vi "get_pixel_number.vi"(11 "Device details":T1={"Device label"="", "Experiment Variable"="", "Variable Value"="", "Pixel"=enum."1"}) -> (2 "Pixel string":string, 3 "Pixel":i32)   [LabVIEW 2018]
uses:
  typedefs/device_details.ctl
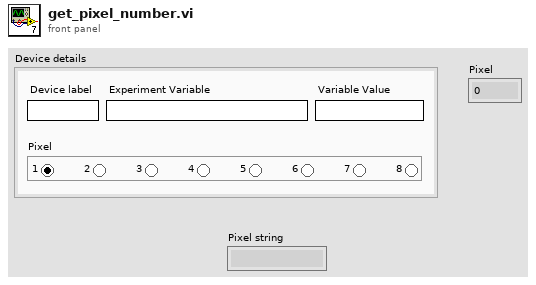
[diagram p1: front panel]
types:
  T1 = typedef "device_details.ctl" = cluster{"Device label":string, "Experiment Variable":string, "Variable Value":string, "Pixel":enum32{"No Selection", "1", "2", "3", "4", "5", "6", "7", "8"}}
  T2 = enum32{"No Selection", "1", "2", "3", "4", "5", "6", "7", "8"}
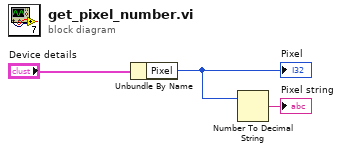
[diagram p0: block diagram]
diagram:
  n1 = Unbundle By Name("Device details") -> ("Pixel"=w1:T2)
  "Pixel" <- w1
  n2 = Number To Decimal String(number=w1) -> (decimal integer string=→"Pixel string":string)  [unwired: 1 in]
